vi "GV_DrawHorArrow.vi"(6 "Color":u32(colorbox), 8 "Vertical":i32, 9 "Right":i32, 10 "Left":i32, 11 "Pict-in":picture) -> (3 "Pict-out":picture)   [LabVIEW 2020, in "Sgraph_lib_V1.lvlib" / "Gviewer.lvclass"]
doc: "Draw Horizontal Arrow"
uses:
  Gviewer.lvclass
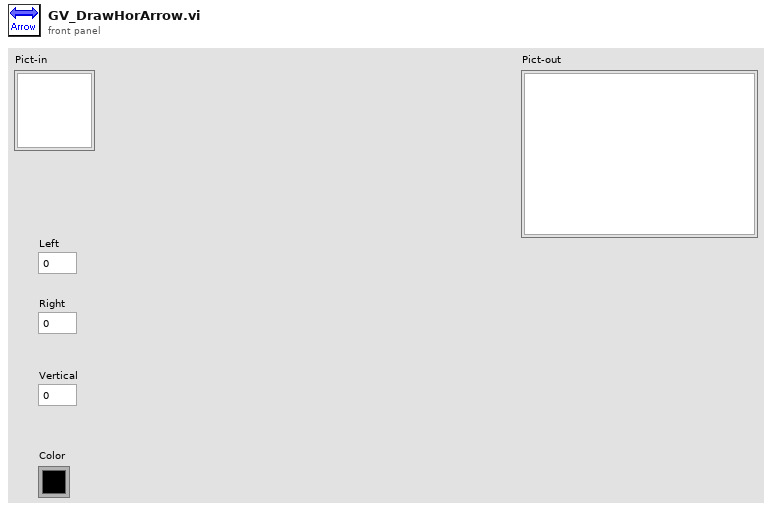
[diagram p1: front panel]
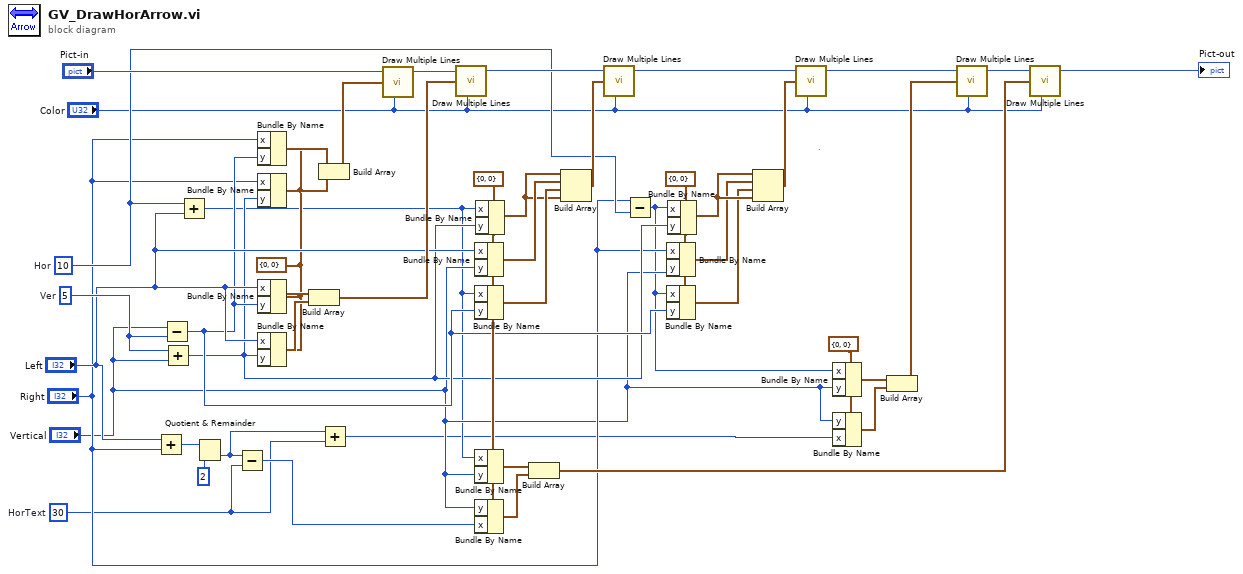
[diagram p0: block diagram]
diagram:
  w9 = cluster{"x":i16, "y":i16} {"x"=0, "y"=0}
  w23 = cluster{"x":i16, "y":i16} {"x"=0, "y"=0}
  w3 = i16 30  # HorText
  w32 = cluster{"x":i16, "y":i16} {"x"=0, "y"=0}
  w47 = i16 5  # Ver
  w17 = i16 10  # Hor
  w24 = cluster{"x":i16, "y":i16} {"x"=0, "y"=0}
  # "`"
  n1 = Add(x="Left", y="Right") -> (x+y=w36:i32)
  n2 = Subtract(x="Vertical", y=w47) -> (x-y=w16:i32)
  n3 = Add(x=w47, y="Vertical") -> (x+y=w15:i32)
  n4 = Add(x=w17, y="Left") -> (x+y=w6:i32)
  n5 = Quotient & Remainder(x=w36, y=2) -> (floor(x/y)=w4:i32)  [unwired: 1 out]
  n6 = Subtract(x=w4, y=w3) -> (x-y=w33:i32)
  n7 = Bundle By Name(cluster=w24, "x"="Right", "y"=w16) -> (w26:cluster{"x":i16, "y":i16})
  n8 = Bundle By Name(cluster=w24, "x"="Right", "y"=w15) -> (w25:cluster{"x":i16, "y":i16})
  n9 = Bundle By Name(cluster=w24, "x"="Left", "y"=w16) -> (w46:cluster{"x":i16, "y":i16})
  n10 = Bundle By Name(cluster=w24, "x"="Left", "y"=w15) -> (w45:cluster{"x":i16, "y":i16})
  n11 = Build Array(w46, w45) -> (w44:cluster{"x":i16, "y":i16}[])
  n12 = Build Array(w26, w25) -> (w27:cluster{"x":i16, "y":i16}[])
  n13 = Add(x=w4, y=w3) -> (x+y=w2:i32)
  n14 = call <vilib>:"Draw Multiple Lines.vi"("picture"="Pict-in", "line endpoints"=w27, "color(black)"="Color") -> ("new picture"=w28:picture)  [unwired: 6 in]
  n15 = call <vilib>:"Draw Multiple Lines.vi"("picture"=w28, "line endpoints"=w44, "color(black)"="Color") -> ("new picture"=w43:picture)  [unwired: 6 in]
  n16 = Bundle By Name(cluster=w32, "x"="Left", "y"="Vertical") -> (w41:cluster{"x":i16, "y":i16})
  n17 = Bundle By Name(cluster=w32, "x"=w6, "y"=w16) -> (w40:cluster{"x":i16, "y":i16})
  n18 = Bundle By Name(cluster=w32, "x"=w6, "y"="Vertical") -> (w34:cluster{"x":i16, "y":i16})
  n19 = Bundle By Name(cluster=w32, "y"="Vertical", "x"=w33) -> (w31:cluster{"x":i16, "y":i16})
  n20 = Bundle By Name(cluster=w32, "x"=w6, "y"=w15) -> (w39:cluster{"x":i16, "y":i16})
  n21 = Build Array(w34, w31) -> (w30:cluster{"x":i16, "y":i16}[])
  n22 = Build Array(w39, w41, w40, w39) -> (w42:cluster{"x":i16, "y":i16}[])
  n23 = call <vilib>:"Draw Multiple Lines.vi"("picture"=w43, "line endpoints"=w42, "color(black)"="Color") -> ("new picture"=w18:picture)  [unwired: 6 in]
  n24 = Subtract(x="Right", y=w17) -> (x-y=w5:i32)
  n25 = Bundle By Name(cluster=w23, "x"="Right", "y"="Vertical") -> (w20:cluster{"x":i16, "y":i16})
  n26 = Bundle By Name(cluster=w23, "x"=w5, "y"=w16) -> (w21:cluster{"x":i16, "y":i16})
  n27 = Bundle By Name(cluster=w23, "x"=w5, "y"=w15) -> (w22:cluster{"x":i16, "y":i16})
  n28 = Build Array(w22, w20, w21, w22) -> (w19:cluster{"x":i16, "y":i16}[])
  n29 = call <vilib>:"Draw Multiple Lines.vi"("picture"=w18, "line endpoints"=w19, "color(black)"="Color") -> ("new picture"=w13:picture)  [unwired: 6 in]
  n30 = Bundle By Name(cluster=w9, "x"=w5, "y"="Vertical") -> (w10:cluster{"x":i16, "y":i16})
  n31 = Bundle By Name(cluster=w9, "y"="Vertical", "x"=w2) -> (w11:cluster{"x":i16, "y":i16})
  n32 = Build Array(w10, w11) -> (w8:cluster{"x":i16, "y":i16}[])
  n33 = call <vilib>:"Draw Multiple Lines.vi"("picture"=w13, "line endpoints"=w8, "color(black)"="Color") -> ("new picture"=w12:picture)  [unwired: 6 in]
  n34 = call <vilib>:"Draw Multiple Lines.vi"("picture"=w12, "line endpoints"=w30, "color(black)"="Color") -> ("new picture"=→"Pict-out":picture)  [unwired: 6 in]
